vi "[V] SC Update.vi"(8 "error in (no error)":errorcluster, 11 "Interface of [V] Sys Cfg in":refnum<class "Interface of [V] Sys Cfg.lvclass">) -> (0 "error out":errorcluster, 3 "Interface of [V] Sys Cfg out":refnum<class "Interface of [V] Sys Cfg.lvclass">)   [LabVIEW 2023, in "[V] Sys Cfg Main.lvlib" / "Interface of [V] Sys Cfg.lvclass"]
uses:
  Interface of [V] Sys Cfg.lvclass
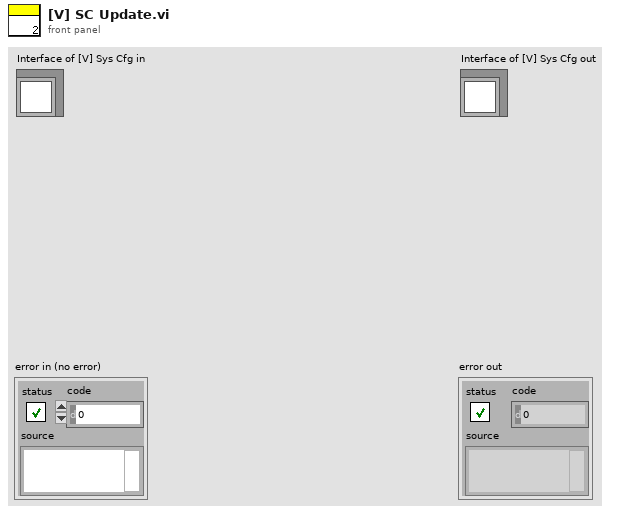
[diagram p1: front panel]
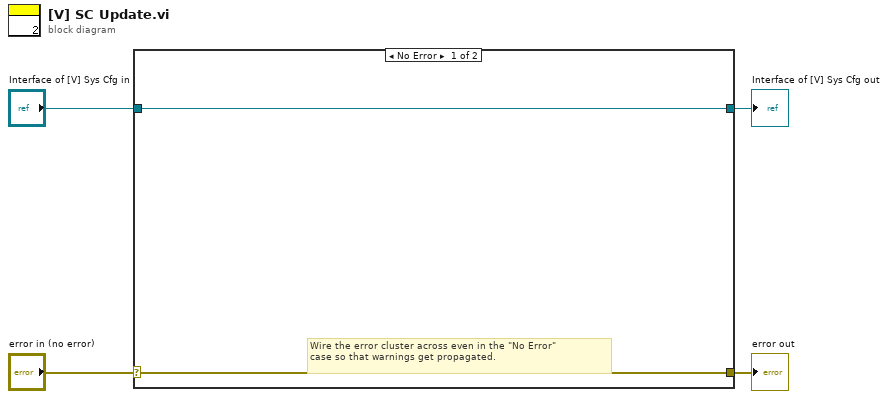
[diagram p0: block diagram]
diagram:
  n1 = case shown="No Error" "error in (no error)" {
    selector: "error in (no error)" -> [w5 w8]
    tunnel: [w5 w8] -> w3
    tunnel: [w6 w7] -> w1
    tunnel: "Interface of [V] Sys Cfg in" -> [w6 w7]
    frame No Error {
      # "Wire the error cluster across even in the \"No Error\"\ncase so that warnings get propagated."
    }
    frame Error {
    }
  }
  "error out" <- w3
  "Interface of [V] Sys Cfg out" <- w1
